vi "Sondenmodell.ParameterUI.vi"() -> ()   [LabVIEW 2016, in "Sondenmodell.lvclass"]
uses:
  Sondenmodell.lvclass
  Package ResourceControl/ViHandler/ViHandler.ViInfo.ctl
  Package Libraries/Message Queue/private/MessageQueue.MessageTypeDef.ctl
  Sondenmodell.lvclass/Sondenmodell.ctl
  Package ErrorHandling/ErrorHandling.lvclass/ErrorHandling.ctl
  Read Sondenmodell.Parameter.vi
  Package ErrorHandling/ErrorHandling.checkForErrorAndHandle.vi
  Package ErrorHandling/ErrorHandling.GetErrorHandler.vi
  Package Libraries/StringFunctions/StringFunctions_ReplaceAllBlindSigns.vi
  <vilib>/dlg_ctls.llb/Space Constant.vi
  <vilib>/Utility/error.llb/Error Cluster From Error Code.vi
  Package Libraries/TimingFunctions/TimingFunctions_getUtcTimestamp.vi
  <vilib>/Utility/error.llb/Trim Whitespace.vi
  <vilib>/Utility/error.llb/Search and Replace Pattern.vi
  Package ErrorHandling/ErrorHandling.addLastErrorToFile.vi
  <vilib>/ErrorRing/Error Ring.xnode
  Package ErrorHandling/ErrorHandling.lvclass
  Package ResourceControl/ViHandler/ViHandler.lvclass
panel:
  in  "Sondenmodell Parameter":T1 {"Erde Masse [kg]" min=0.0 max=10000000.0 format="%#.0f"}
  in  "Model Path":path
  out "Sondenmodell":refnum<data-value>
  out "ViInfoTemp":T2
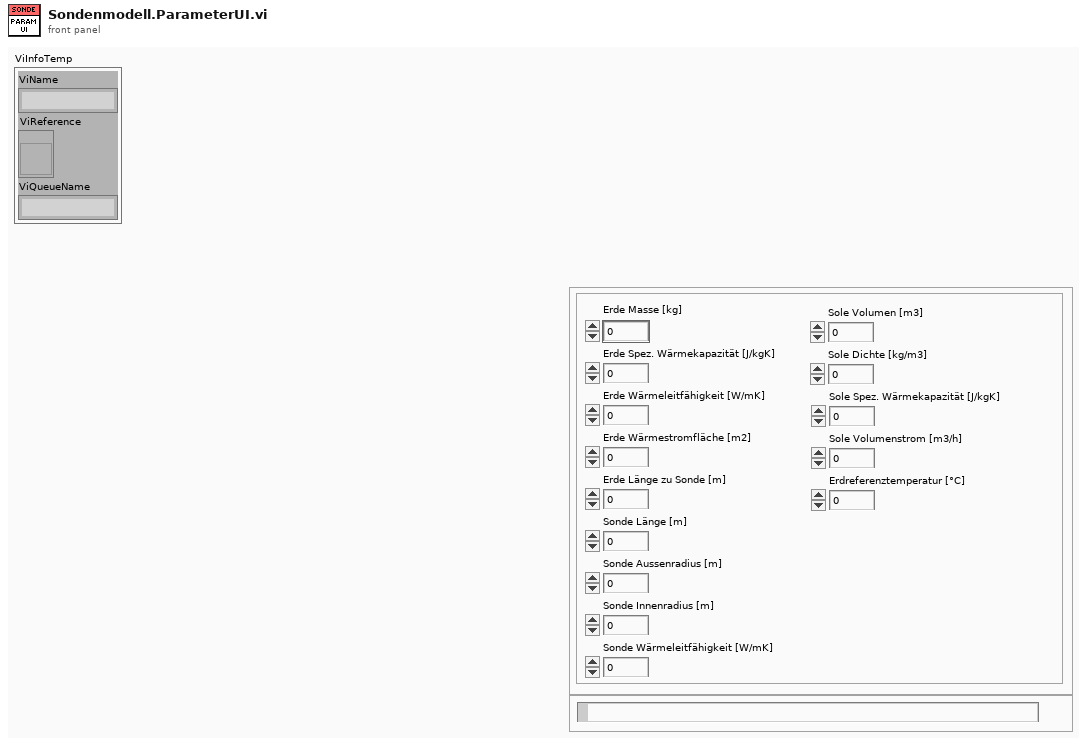
[diagram p1: front panel]
types:
  T1 = cluster{"Erde Masse [kg]":dbl, "Erde Spez. Wärmekapazität [J/kgK]":dbl, "Erde Wärmeleitfähigkeit [W/mK]":dbl, "Erde Wärmestromfläche [m2]":dbl, "Erde Länge zu Sonde [m]":dbl, "Sonde Länge [m]":dbl, "Sonde Aussenradius [m]":dbl, "Sonde Innenradius [m]":dbl, "Sonde Wärmeleitfähigkeit [W/mK]":dbl, "Sole Volumen [m3]":dbl, "Sole Dichte [kg/m3]":dbl, "Sole Spez. Wärmekapazität [J/kgK]":dbl, "Sole Volumenstrom [m3/h]":dbl, "Erdreferenztemperatur [°C]":dbl}
  T2 = typedef "ViHandler.lvclass/ViHandler.ViInfo.ctl" = cluster{"ViName":string, "ViReference":refnum<vi>, "ViQueueName":string}
  T3 = typedef "MessageQueue.MessageTypeDef.ctl" = cluster{"Message":string, "Data":variant}
  T4 = enum16{"open", "replace", "create", "open or create", "replace or create", "replace or create with confirmation"}
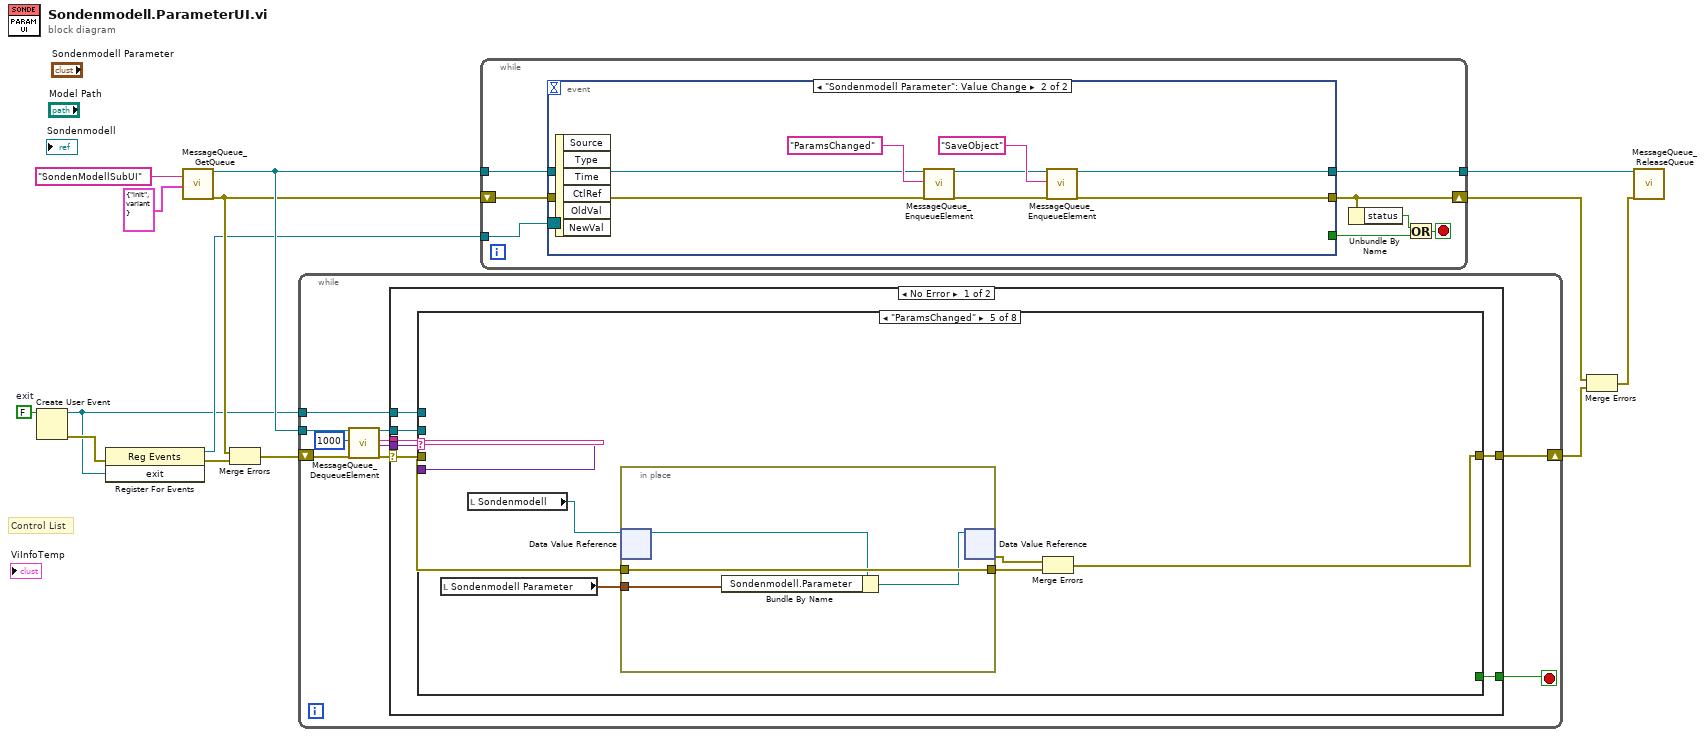
[diagram p0: block diagram]
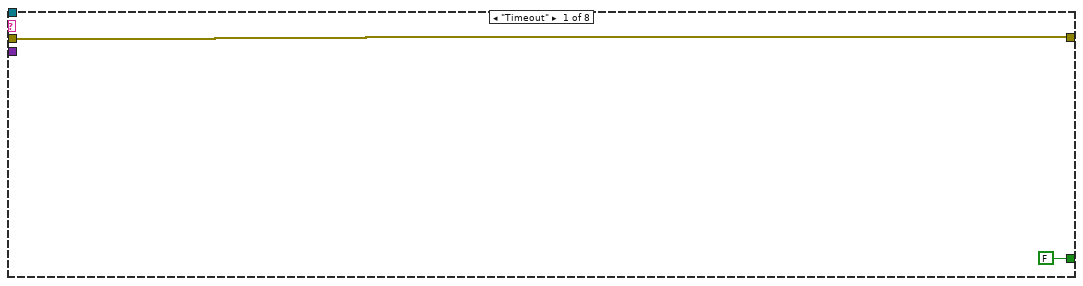
[diagram p2: hidden frame]
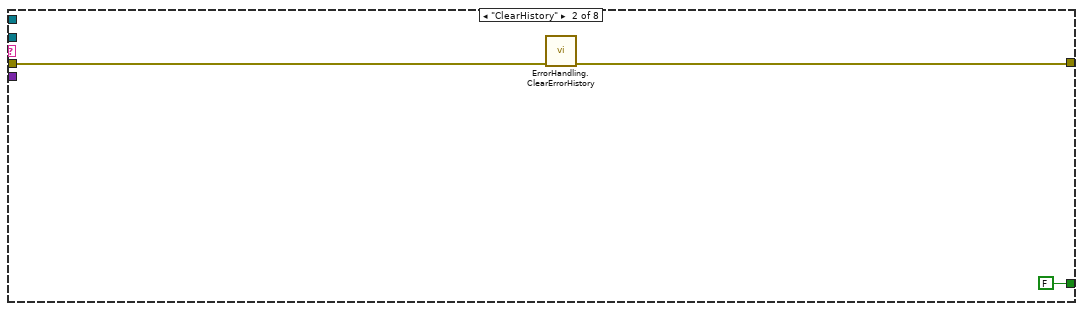
[diagram p3: hidden frame]
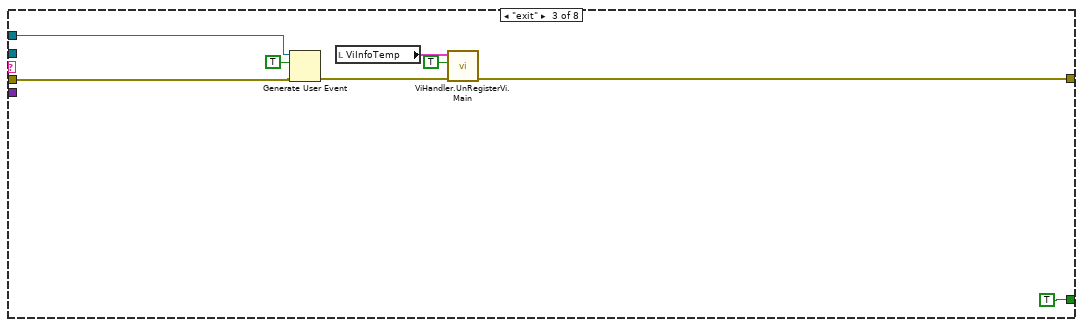
[diagram p4: hidden frame]
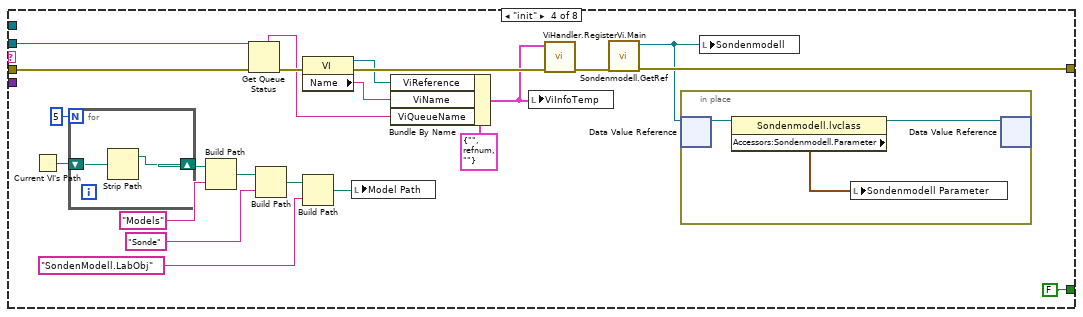
[diagram p5: hidden frame]
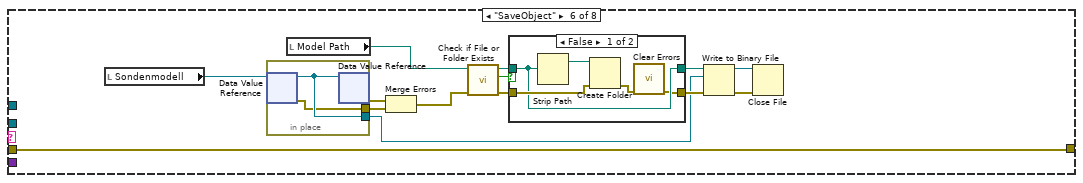
[diagram p6: hidden frame]
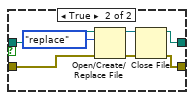
[diagram p7: hidden frame]
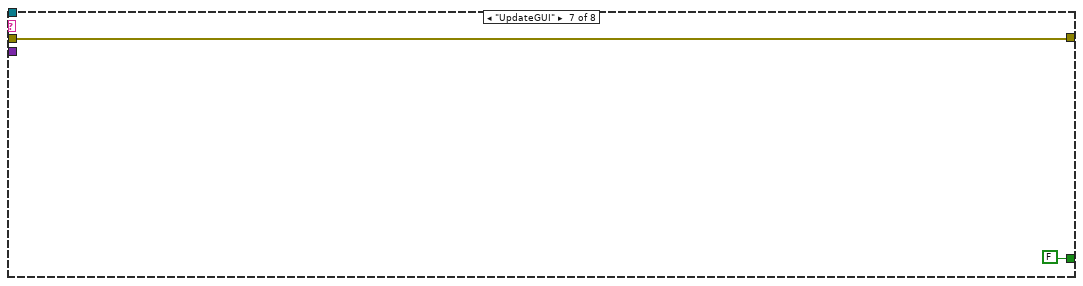
[diagram p8: hidden frame]
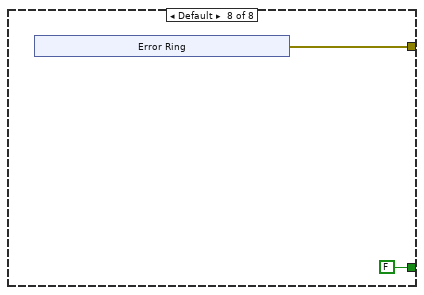
[diagram p9: hidden frame]
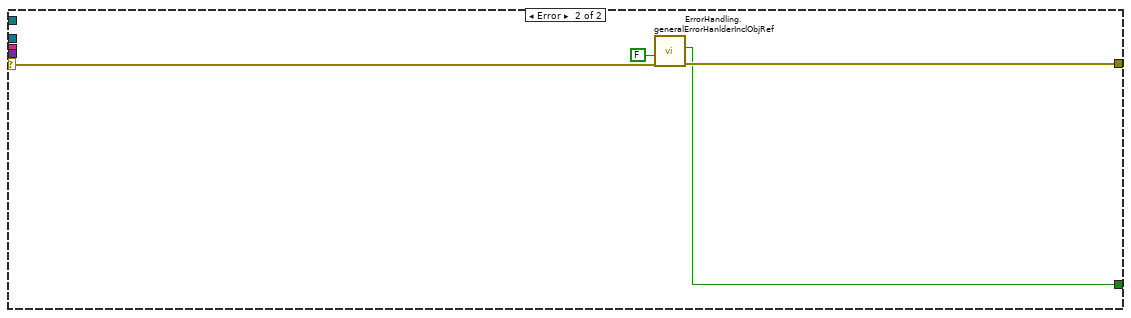
[diagram p10: hidden frame]
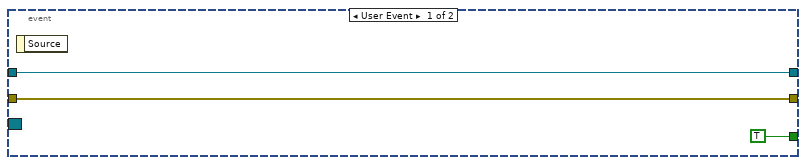
[diagram p11: hidden frame]
diagram:
  w7 = FALSE  # exit
  # "Control List"
  n1 = Create User Event(user event datatype=w7) -> (user event=w5:refnum<user-event>, error out=w6:errorcluster)  [unwired: 1 in]
  n2 = register-events(error in=w6, w5) -> (reference out=w9:refnum<event-registration>, error out=w11:errorcluster)  [unwired: 1 in]
  n3 = call "MessageQueue_GetQueue.vi"("Name"="SondenModellSubUI", "OptionalInitValue"=T3 {"Message"="init", "Data"=variant}) -> ("QueueOut"=w13:refnum<queue>, "ErrorOut"=w10:errorcluster)  [unwired: 15 in, 1 out]
  n4 = Merge Errors(w10, w11) -> (w8:errorcluster)
  n5 = while {
    tunnel: w13 -> [w24]
    tunnel: w5 -> [w17]
    shift-right: [w16] -> w3
    shift-left: w8 -> [w18]
    stop <- w19 stop-if-true
    n6 = call "MessageQueue_DequeueElement.vi"("QueueIn"=w24, "Timeout"=1000, "ErrorIn"=w18) -> ("QueueOut"=w22:refnum<queue>, "Message"=w21:string, "Data"=w20:variant, "ErrorOut"=w23:errorcluster)  [unwired: 12 in, 1 out]
    n7 = case shown="No Error" w23 {
      selector: w23 -> [w27 w122]
      tunnel: w22 -> [w31 _]
      tunnel: w21 -> [w30 _]
      tunnel: w20 -> [w29 _]
      tunnel: [w28 w120] -> w19
      tunnel: w17 -> [w26 _]
      tunnel: [w25 w121] -> w16
      frame No Error {
        n8 = case shown="\"ParamsChanged\"" w30 {
          tunnel: w31 -> [_ _ _ w60 _ _ _ _]
          tunnel: w29 -> [_ _ _ _ _ _ _ _]
          tunnel: [FALSE FALSE TRUE FALSE _ _ FALSE FALSE] -> w28
          tunnel: w27 -> [w32 w35 w42 w57 w74 w95 w110 _]
          tunnel: w26 -> [_ _ w41 _ _ _ _ _]
          tunnel: [w32 w34 w38 w55 w73 w95 w110 w113] -> w25
          frame "Timeout" {
          }
          frame "ClearHistory" {
            n9 = call "ErrorHandling.ClearErrorHistory.vi"("error IO"=w35) -> ("error IO"=w34:errorcluster)  [unwired: 10 in]
          }
          frame "exit" {
            n10 = Generate User Event(user event=w41, event data cluster=TRUE ("event data"), error in=w42) -> (error out=w39:errorcluster)  [unwired: 1 in, 1 out]
            n11 = local read "ViInfoTemp"() -> (w40:T2)
            n12 = call "ViHandler.UnRegisterVi.Main.vi"("ErrorIn"=w39, "FinalExit?"=TRUE, "ViInfo"=w40) -> ("ErrorOut"=w38:errorcluster)  [unwired: 7 in, 1 out]
          }
          frame "init" {
            n13 = Current VI's Path() -> (path=w46:path)
            n14 = for {
              N: 5 -> [_]
              shift-right: [w67] -> w53
              shift-left: w46 -> [w68]
              n15 = Strip Path(path=w68) -> (stripped path=w67:path)  [unwired: 1 out]
            }
            n16 = Build Path(base path=w53, name or relative path="Models") -> (appended path=w51:path)
            n17 = Get Queue Status(queue=w60, error in (no error)=w57) -> (queue name=w58:string, error out=w64:errorcluster)  [unwired: 1 in, 6 out]
            n18 = Build Path(base path=w51, name or relative path="Sonde") -> (appended path=w49:path)
            n19 = property class="VI"(error in=w64) -> (reference out=w62:refnum<vi>, error out=w63:errorcluster, "Name"=w61:string)  [unwired: 1 in]
            n20 = Build Path(base path=w49, name or relative path="SondenModell.LabObj") -> (appended path=w48:path)
            n21 = local write "Model Path"(w48) -> ()
            n22 = Bundle By Name(cluster=T2 {"ViName"="", "ViReference"=refnum, "ViQueueName"=""} ("ViInfo"), "ViReference"=w62, "ViName"=w61, "ViQueueName"=w58) -> (w59:T2)
            n23 = local write "ViInfoTemp"(w59) -> ()
            n24 = call "ViHandler.RegisterVi.Main.vi"("ErrorIn"=w63, "ViInfo"=w59) -> ("ErrorOut"=w56:errorcluster)  [unwired: 9 in]
            n25 = call "Sondenmodell.GetRef.vi"("Error In"=w56) -> ("Error out"=w55:errorcluster, "Sondenmodell"=w45:refnum<data-value>)  [unwired: 9 in]
            n26 = in-place {
              n27 = in-place-dvr #1(w45) -> (w71:refnum<class "Sondenmodell.lvclass">)  [unwired: 1 out]
              n28 = property class="Sondenmodell.lvclass"(reference=w71) -> (reference out=w70:refnum<class "Sondenmodell.lvclass">, "Accessors:Sondenmodell.Parameter"=w69:T1)  [unwired: 1 in, 1 out]
              n29 = local write "Sondenmodell Parameter"(w69) -> ()
              n30 = in-place-dvr #1(w70) -> ()  [unwired: 2 out]
            }
            n31 = local write "Sondenmodell"(w45) -> ()
          }
          frame "ParamsChanged" {
            n32 = local read "Sondenmodell Parameter"() -> (w77:T1)
            n33 = local read "Sondenmodell"() -> (w72:refnum<data-value>)
            n34 = in-place {
              in-place-border: w77 -> [w81]
              in-place-border: w74 -> [w80]
              in-place-border: [w80] -> w75
              n35 = in-place-dvr #2(w72) -> (w79:refnum<class "Sondenmodell.lvclass">)  [unwired: 1 out]
              n36 = Bundle By Name(cluster=w79, "Sondenmodell.Parameter"=w81) -> (w78:refnum<class "Sondenmodell.lvclass">)
              n37 = in-place-dvr #2(w78) -> (w76:errorcluster)  [unwired: 1 out]
            }
            n38 = Merge Errors(w76, w75) -> (w73:errorcluster)
          }
          frame "SaveObject" {
            n39 = local read "Sondenmodell"() -> (w82:refnum<data-value>)
            n40 = in-place {
              in-place-border: [w97] -> w83
              in-place-border: [w96] -> w87
              n41 = in-place-dvr #3(w82) -> (w97:refnum<class "Sondenmodell.lvclass">, w96:errorcluster)
              n42 = in-place-dvr #3(w97) -> (w86:errorcluster)  [unwired: 1 out]
            }
            n43 = local read "Model Path"() -> (w84:path)
            n44 = Merge Errors(w86, w87) -> (w85:errorcluster)
            n45 = call <vilib>:"Check if File or Folder Exists.vi"("error in (no error)"=w85, "path"=w84) -> ("error out"=w92:errorcluster, "file or folder exists?"=w94:bool, "dup path"=w93:path)  [unwired: 7 in]
            n46 = case shown="False" w94 {
              tunnel: w93 -> [w100 w109]
              tunnel: [w100 w105] -> w91
              tunnel: w92 -> [w101 w108]
              tunnel: [w98 w104] -> w90
              frame False {
                n47 = Strip Path(path=w100) -> (stripped path=w102:path)  [unwired: 1 out]
                n48 = Create Folder(path (use dialog)=w102, error in=w101) -> (error out=w99:errorcluster)  [unwired: 1 in, 2 out]
                n49 = call <vilib>:"Clear Errors.vi"("error in (no error)"=w99) -> ("error out"=w98:errorcluster)  [unwired: 5 in, 1 out]
              }
              frame True {
                n50 = Open/Create/Replace File(file path (use dialog)=w109, error in=w108, operation (0:open)=T4."replace") -> (refnum out=w106:refnum<file>, error out=w103:errorcluster)  [unwired: 3 in, 1 out]
                n51 = Close File(refnum=w106, error in=w103) -> (path=w105:path, error out=w104:errorcluster)
              }
            }
            n52 = Write to Binary File(file (use dialog)=w91, data=w83, error in=w90) -> (refnum out=w88:refnum<file>, error out=w89:errorcluster)  [unwired: 3 in, 1 out]
            n53 = Close File(refnum=w88, error in=w89) -> ()  [unwired: 2 out]
          }
          frame "UpdateGUI" {
          }
          frame Default {
            n54 = xnode "Error Ring"() -> ("error out"=w113:errorcluster)
          }
        }
      }
      frame Error {
        n55 = call "ErrorHandling.generalErrorHanlderInclObjRef.vi"("error in"=w122, "StopOnError"=FALSE) -> ("error out"=w121:errorcluster, "Stop"=w120:bool)  [unwired: 7 in, 1 out]
      }
    }
  }
  n56 = while {
    tunnel: w13 -> [w130]
    tunnel: [w129] -> w14
    shift-right: [w126] -> w2
    shift-left: w10 -> [w128]
    tunnel: w9 -> [w123]
    stop <- w125 stop-if-true
    n57 = event shown="[1] \"Sondenmodell Parameter\": Value Change" {
      selector: w123 -> [_ _]
      dyn-events: _ -> [_ _]
      timeout: _ -> [_ _]
      tunnel: w130 -> [w132 w134]
      tunnel: [w132 w135] -> w129
      tunnel: [w131 w136] -> w126
      tunnel: w128 -> [w131 w137]
      tunnel: [TRUE _] -> w127
      event User Event {
        n58 = event-data() -> ()  [unwired: 1 in, 1 out]
      }
      event "Sondenmodell Parameter": Value Change {
        n59 = event-data() -> ()  [unwired: 1 in, 6 out]
        n60 = call "MessageQueue_EnqueueElement.vi"("QueueIn"=w134, "Message"="ParamsChanged", "ErrorIn"=w137) -> ("QueueOut"=w139:refnum<queue>, "ErrorOut"=w138:errorcluster)  [unwired: 15 in]
        n61 = call "MessageQueue_EnqueueElement.vi"("QueueIn"=w139, "Message"="SaveObject", "ErrorIn"=w138) -> ("QueueOut"=w135:refnum<queue>, "ErrorOut"=w136:errorcluster)  [unwired: 15 in]
      }
    }
    n62 = Unbundle By Name(w126) -> ("status"=w124:bool)
    n63 = Or(x=w124, y=w127) -> (x .or. y?=w125:bool)
  }
  n64 = Merge Errors(w2, w3) -> (w1:errorcluster)
  n65 = call "MessageQueue_ReleaseQueue.vi"("QueueIn"=w14, "ErrorIn"=w1) -> ()  [unwired: 15 in, 3 out]
